vi "菜单-下载.vi"(8 "error in (no error)":errorcluster caption="错误输入（无错误）", 11 "程序响应 输入":refnum<class "程序响应.lvclass">) -> (0 "error out":errorcluster caption="错误输出", 3 "程序响应 输出":refnum<class "程序响应.lvclass">)   [LabVIEW 2018, in "程序响应.lvlib" / "程序响应.lvclass"]
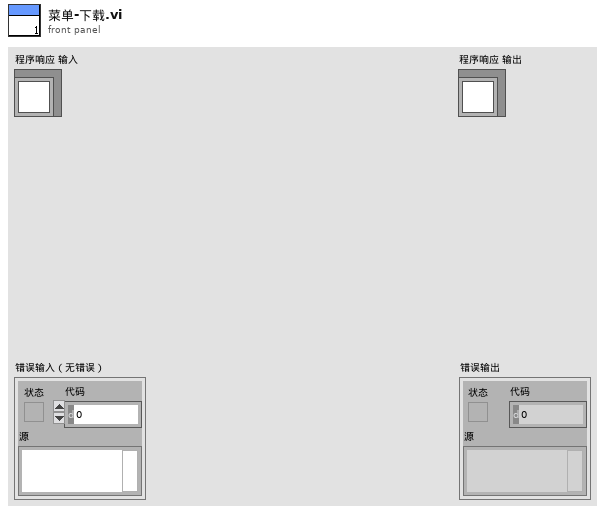
[diagram p1: front panel]
types:
  T1 = enum16{"open", "replace", "create", "open or create", "replace or create", "replace or create with confirmation"}
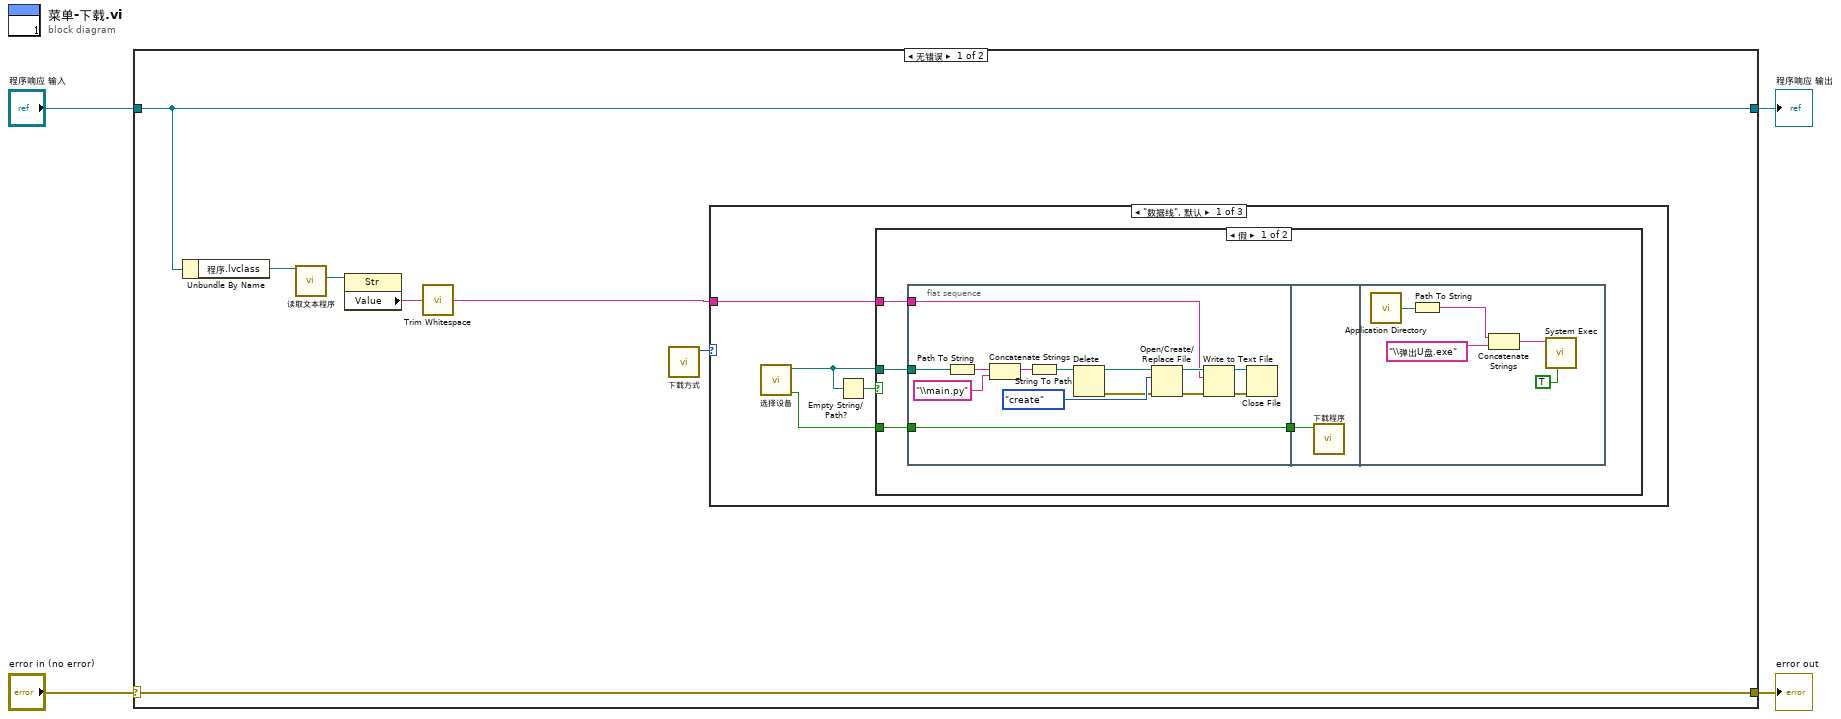
[diagram p0: block diagram]
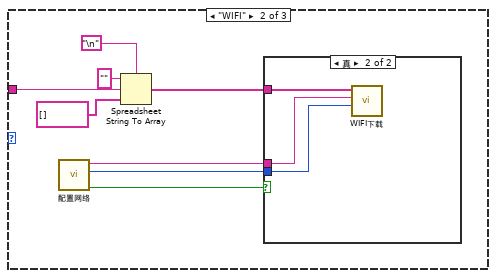
[diagram p3: hidden frame]
diagram:
  n1 = case shown="无错误" "error in (no error)" {
    selector: "error in (no error)" -> [w11 w52]
    tunnel: [w11 w52] -> w3
    tunnel: [w10 w51] -> w1
    tunnel: "程序响应 输入" -> [w10 w51]
    frame No Error {
      n2 = Unbundle By Name(w10) -> ("程序.lvclass"=w9:refnum<class "程序.lvclass">)
      n3 = call-dynamic "读取文本程序.vi"("程序输入"=w9) -> ("文本程序"=w8:refnum<vi>)  [unwired: 8 in, 2 out]
      n4 = property class="Str"(reference=w8) -> ("Value"=w6:string)  [unwired: 1 in, 2 out]
      n5 = call <vilib>:"Trim Whitespace.vi"("string"=w6) -> ("trimmed string"=w5:string)  [unwired: 1 in]
      n6 = call "下载方式.vi"() -> ("下载方式"=w7:enum32{"数据线", "WIFI", "取消"})  [unwired: 11 in]
      n7 = case shown="\"数据线\", 默认" w7 {
        tunnel: w5 -> [w15 w47 _]
        frame "数据线", Default {
          n8 = call "选择设备.vi"() -> ("boot?"=w12:bool, "路径"=w14:path)  [unwired: 10 in]
          n9 = Empty String/Path?(string/path=w14) -> (empty?=w13:bool)
          n10 = case shown="假" w13 {
            tunnel: w14 -> [w18 _]
            tunnel: w15 -> [w19 _]
            tunnel: w12 -> [w17 _]
            frame False {
              n11 = flat-sequence {
                tunnel: w19 -> [w28]
                tunnel: w18 -> [w27]
                tunnel: w17 -> [w20]
                tunnel: [w20] -> w16
                tunnel: w16 -> [w34]
                frame #0 {
                  n12 = Path To String(path=w27) -> (string=w24:string)
                  n13 = Concatenate Strings(w24, "\\main.py" ("名称或相对路径")) -> (w25:string)
                  n14 = String To Path(string=w25) -> (path=w23:path)
                  n15 = Delete(path (use dialog)=w23) -> (deleted path=w22:path, error out=w21:errorcluster)  [unwired: 4 in, 1 out]
                  n16 = Open/Create/Replace File(file path (use dialog)=w22, error in=w21, operation (0:open)=T1."create" ("操作(0:open)")) -> (refnum out=w33:refnum<file>, error out=w32:errorcluster)  [unwired: 3 in, 1 out]
                  n17 = Write to Text File(file (use dialog)=w33, text=w28, error in=w32) -> (refnum out=w31:refnum<file>, error out=w30:errorcluster)  [unwired: 1 in, 1 out]
                  n18 = Close File(refnum=w31, error in=w30) -> ()  [unwired: 2 out]
                }
                frame #1 {
                  n19 = call "下载程序.vi"("boot?"=w34) -> ()  [unwired: 11 in]
                }
                frame #2 {
                  n20 = call <vilib>:"Application Directory.vi"() -> ("Application Directory"=w39:path)
                  n21 = Path To String(path=w39) -> (string=w36:string)
                  n22 = Concatenate Strings(w36, "\\弹出U盘.exe" ("字符串")) -> (w37:string)
                  n23 = call <vilib>:"System Exec.vi"("run minimized? (F)"=TRUE, "command line"=w37) -> ()  [unwired: 6 in, 4 out]
                }
              }
            }
            frame True {
            }
          }
        }
        frame "WIFI" {
          n24 = call "配置网络.vi"() -> ("下载"=w40:bool, "端口号"=w41:u16, "IP"=w42:string)  [unwired: 9 in]
          n25 = Spreadsheet String To Array(delimiter (Tab)="\n", format string="" ("格式字符串"), spreadsheet string=w47, array type (2D Dbl)=string[] []) -> (array=w43:string[])
          n26 = case shown="真" w40 {
            tunnel: w43 -> [_ w50]
            tunnel: w42 -> [_ w49]
            tunnel: w41 -> [_ w48]
            frame False {
            }
            frame True {
              n27 = call "WIFI下载.vi"("远程端口"=w48, "地址"=w49, "程序"=w50) -> ()  [unwired: 9 in]
            }
          }
        }
        frame "取消" {
        }
      }
    }
    frame Error {
    }
  }
  "error out" <- w3
  "程序响应 输出" <- w1
